vi "Peek Content.vi"(8 "Error In":errorcluster, 11 "Parser In":refnum<class "Lexer.lvclass">) -> (0 "Error Out":errorcluster, 2 "Character":string, 3 "Parser Out":refnum<class "Lexer.lvclass">)   [LabVIEW 2018, in "Toolkit.lvlib" / "Lexer.lvclass"]
uses:
  Lexer.lvclass
  Lexer.lvclass/Lexer.ctl
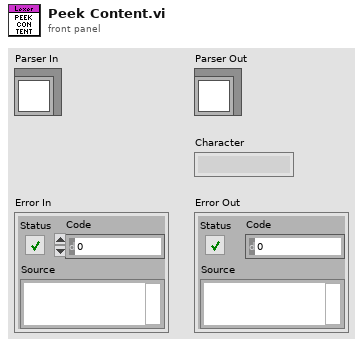
[diagram p1: front panel]
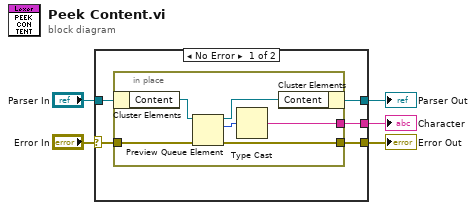
[diagram p0: block diagram]
diagram:
  n1 = case shown="No Error" "Error In" {
    selector: "Error In" -> [w6 w17]
    tunnel: [w10 w17] -> w5
    tunnel: [w9 w18] -> w4
    tunnel: "Parser In" -> [w8 w18]
    tunnel: [w7 _] -> w2
    frame No Error {
      n2 = in-place {
        in-place-border: w6 -> [w14]
        in-place-border: [w13] -> w10
        in-place-border: [w11] -> w7
        n3 = in-place-cluster #1(w8) -> ("Content"=w16:refnum<queue>)
        n4 = Preview Queue Element(queue=w16, error in (no error)=w14) -> (queue out=w15:refnum<queue>, element=w12:u8, error out=w13:errorcluster)  [unwired: 1 in, 1 out]
        n5 = Type Cast(x=w12) -> (*(type *) &x=w11:string)  [unwired: 1 in]
        n6 = in-place-cluster #1("Content"=w15) -> (w9:refnum<class "Lexer.lvclass">)
      }
    }
    frame Error {
    }
  }
  "Error Out" <- w5
  "Parser Out" <- w4
  "Character" <- w2
